vi "Initialize Hardware.vi"(8 "error in":errorcluster, 11 "device parameters":T3) -> (0 "error out":errorcluster, 3 "RT handles":T2, 5 "board_info":T1 {"capability_flags" format="%.0x"; "serial" format="%.0x"})   [LabVIEW 2020, in "AIM ARINC 429 Engine.lvlib" / "Custom Device.lvlib"]
uses:
  Custom Device.lvlib
  Shared/Device Parameters.ctl
  Hardware Handles.ctl
  Hardware API/AIM ARINC 429 Hardware API.lvlib
  <instrlib>/AIM GmbH/ARINC-429/AIM429LV.lvlib
  <instrlib>/AIM GmbH/ARINC-429/VIs/TypeDefinitions/Board_Info.ctl
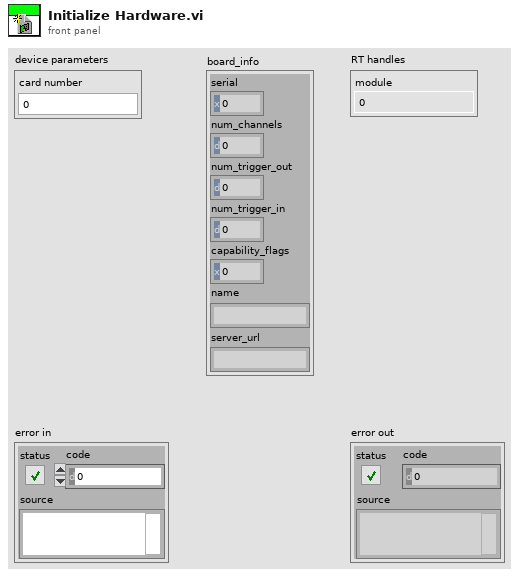
[diagram p1: front panel]
types:
  T1 = typedef "AIM429LV.lvlib/Board_Info.ctl" = cluster{"serial":u32, "num_channels":u32, "num_trigger_out":u32, "num_trigger_in":u32, "capability_flags":u32, "name":string, "server_url":string}
  T2 = typedef "AIM ARINC 429 Engine.lvlib/Custom Device.lvlib/Hardware Handles.ctl" = cluster{"module":u8}
  T3 = typedef "Device Parameters.ctl" = cluster{"card number":u8}
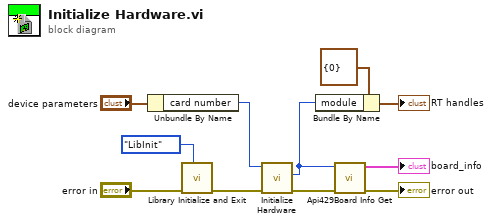
[diagram p0: block diagram]
diagram:
  n1 = Unbundle By Name("device parameters") -> ("card number"=w5:u8)
  n2 = call "Library Initialize and Exit.vi"("action"=enum16{"LibInit", "LibExit"}."LibInit", "error in"="error in") -> ("error out"=w6:errorcluster)  [unwired: 7 in, 2 out]
  n3 = call "Initialize Hardware.vi"("error in"=w6, "board identifier in"=w5) -> ("error out"=w3:errorcluster, "module handle out"=w4:u8)  [unwired: 7 in, 1 out]
  n4 = Bundle By Name(cluster=T2 {"module"=0} ("RT handles"), "module"=w4) -> (→"RT handles":T2)
  n5 = call <instrlib>:"Api429Board Info Get.vi"("error in (no error)"=w3, "board_handle"=w4) -> ("error out"=→"error out":errorcluster, "board_info"=→"board_info":T1)  [unwired: 8 in]
